vi "StartData.vi"(8 "error in (no error)":errorcluster, 11 "Class In":refnum<class "C37.118 Sim.lvclass">) -> (0 "error out":errorcluster, 3 "Class Out":refnum<class "C37.118 Sim.lvclass">)   [LabVIEW 2018, in "SensorPlugins.lvlib" / "C37.118 Sim.lvclass"]
uses:
  C37.118 Sim.lvclass
  X:/Projects/PMUCal/Modules/Sensor/SensorPlugins/PmuBaseClass/PmuBase.lvclass
  PmuBaseClass/PmuBase.lvclass/PmuBase.ctl
  C37.118 Sim.lvclass/C37.118 Sim.ctl
  PmuBaseClass/Accessors/Read PmuConfig.vi
  Accessors/Read Function.vi
  Accessors/Write Function.vi
  PmuBaseClass/Accessors/Write PmuConfig.vi
  FGen/MemberClasses/FunctionBaseClass/FunctionBase.lvclass
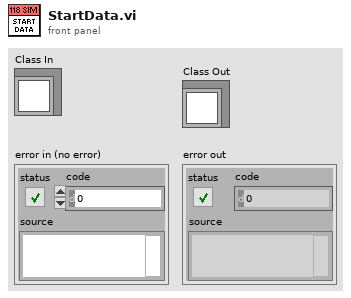
[diagram p1: front panel]
types:
  T1 = typedef "SensorPlugins.lvlib/PmuBase.lvclass/PmuConfig.ctl" = cluster{"Class":enum16{"M", "P"}, "Fs":i32, "F0":i32, "FSamp":i32, "SettlingTime":dbl, "T0":ext}
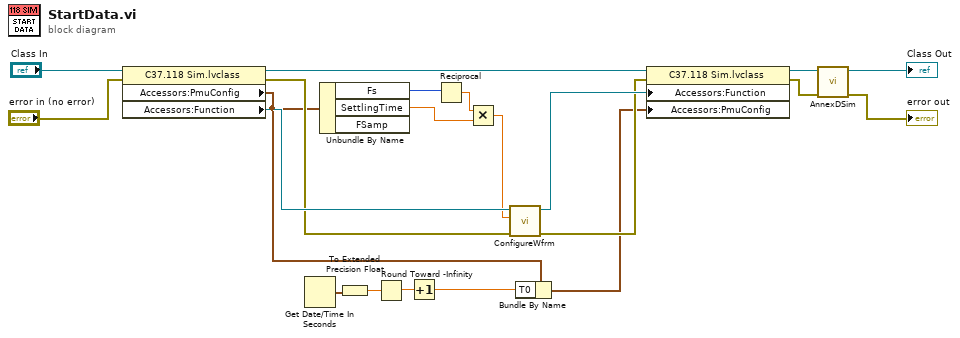
[diagram p0: block diagram]
diagram:
  n1 = property class="C37.118 Sim.lvclass"(reference="Class In", error in="error in (no error)") -> (reference out=w18:refnum<class "C37.118 Sim.lvclass">, error out=w12:errorcluster, "Accessors:PmuConfig"=w6:T1, "Accessors:Function"=w13:refnum<class "FunctionBase.lvclass">)
  n2 = Get Date/Time In Seconds() -> (seconds since 1Jan1904=w5:timestamp)
  n3 = Unbundle By Name(w6) -> ("Fs"=w20:i32, "SettlingTime"=w8:dbl)  [unwired: 1 out]
  n4 = To Extended Precision Float(1:w5) -> (0:w4:ext)
  n5 = Round Toward -Infinity(1:w4) -> (0:w3:ext)
  n6 = Increment(x=w3) -> (x+1=w2:ext)
  n7 = Reciprocal(x=w20) -> (1/x=w9:dbl)
  n8 = Multiply(x=w9, y=w8) -> (x*y=w7:dbl)
  n9 = call-dynamic "ConfigureWfrm.vi"("error in (no error)"=w12, "SampleRate"=w7, "FunctionBase in"=w13) -> ("error out"=w10:errorcluster, "FunctionBase out"=w11:refnum<class "FunctionBase.lvclass">)  [unwired: 7 in]
  n10 = Bundle By Name(cluster=w6, "T0"=w2) -> (w1:T1)
  n11 = property class="C37.118 Sim.lvclass"(reference=w18, error in=w10, "Accessors:Function"=w11, "Accessors:PmuConfig"=w1) -> (reference out=w17:refnum<class "C37.118 Sim.lvclass">, error out=w15:errorcluster)
  n12 = call "AnnexDSim.vi"("error in (no error)"=w15, "C37.118 Sim in"=w17) -> ("error out"=→"error out":errorcluster, "C37.118 Sim out"=→"Class Out":refnum<class "C37.118 Sim.lvclass">)  [unwired: 8 in]
